vi "Find Direct Dependencies.vi"(8 "error in (no error)":errorcluster, 9 "LibraryName":string="ModuleA", 10 "Project Path":path=path "E:/sw-deps-monitor/Source/BuildSpecs/Modules/ModuleA.lvproj") -> (0 "error out":errorcluster, 2 "InDirect ActualDependencies":string[](array[string]), 3 "Direct ActualDependencies":string[](array[string]))   [LabVIEW 2019, in "Hawkeye.lvlib"]
uses:
  Hawkeye.lvlib
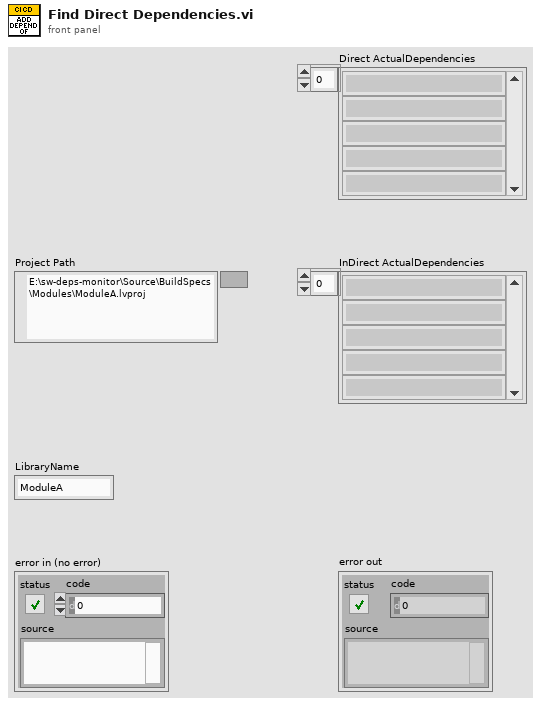
[diagram p1: front panel]
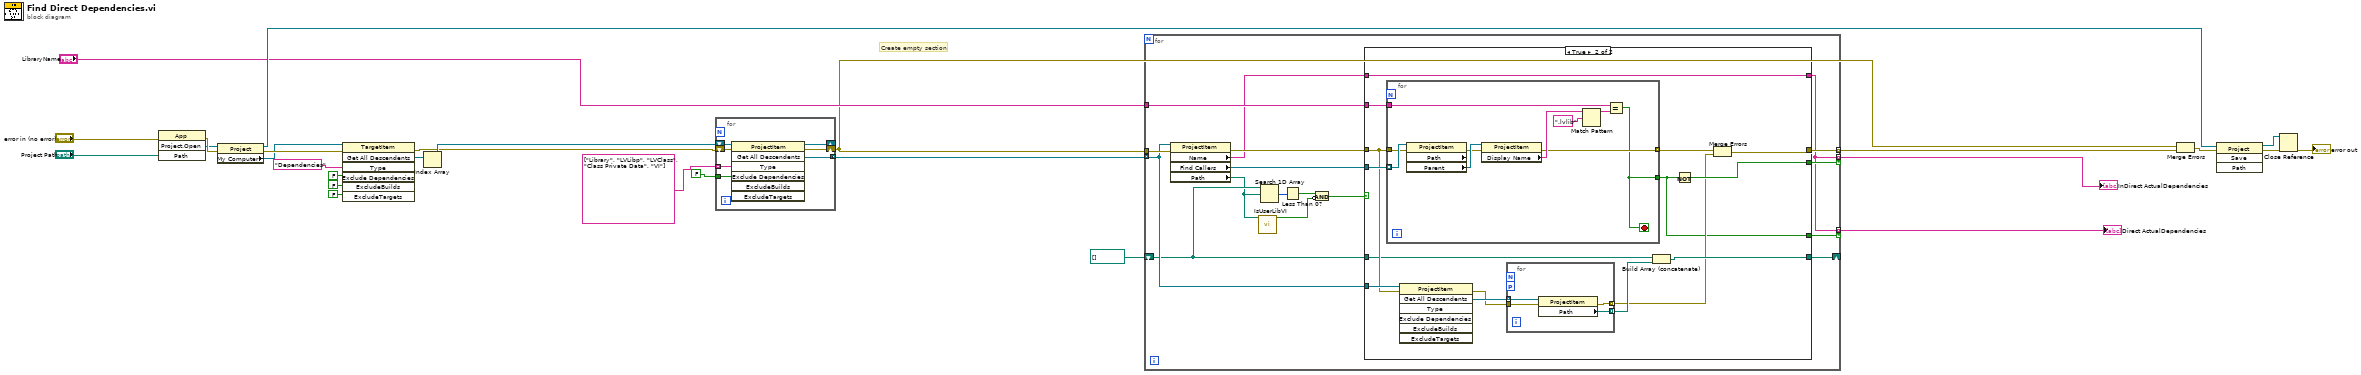
[diagram p0: block diagram]
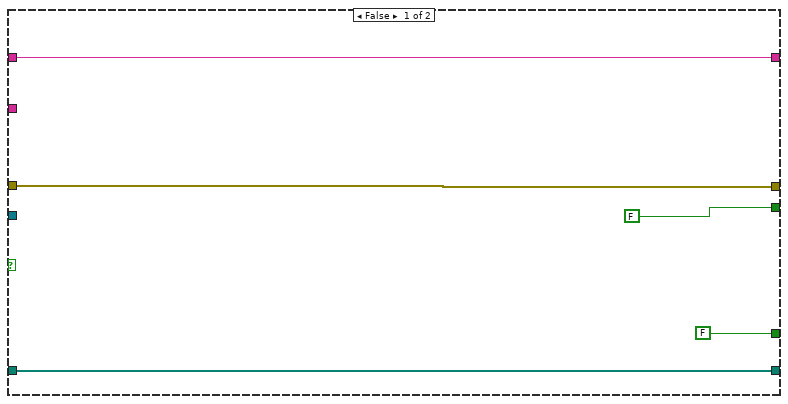
[diagram p2: hidden frame]
diagram:
  # "Create empty section"
  n1 = invoke class="App" method="Project.Open"(error in="error in (no error)", "Path"="Project Path") -> (error out=w26:errorcluster, "Project:Open"=w11:refnum<vi>)  [unwired: 2 in, 2 out]
  n2 = property class="Project"(reference=w11, error in=w26) -> (reference out=w17:refnum<vi>, error out=w20:errorcluster, "My Computer"=w10:refnum<vi>)
  n3 = invoke class="TargetItem" method="Get All Descendents"(reference=w10, error in=w20, "Type"="Dependencies", "Exclude Dependencies"=FALSE ("ExcludeDependencies"), "ExcludeBuilds"=FALSE, "ExcludeTargets"=FALSE) -> (error out=w19:errorcluster, "All Descendents"=w9:refnum<vi>[])  [unwired: 1 in, 5 out]
  n4 = Index Array(array=w9) -> (element=w21:refnum<vi>)  [unwired: 1 in]
  n5 = for {
    shift-right: [w33] -> _
    shift-left: w21 -> [w34]
    shift-right: [w31] -> w5
    shift-left: w19 -> [w32]
    tunnel: FALSE ("ExcludeDependencies") -> [w28]
    tunnel: string[] ["Library", "LVLibp", "LVClass", "Class Private Data", "VI"] ("Type") -> [w30] mode=indexing
    tunnel: [w29] -> w2 mode=concatenating
    n6 = invoke class="ProjectItem" method="Get All Descendents"(reference=w34, error in=w32, "Type"=w30, "Exclude Dependencies"=w28) -> (reference out=w33:refnum<vi>, error out=w31:errorcluster, "All Descendents"=w29:refnum<vi>[])  [unwired: 3 in, 4 out]
  }
  n7 = for {
    tunnel: w5 -> [w51]
    tunnel: w2 -> [w44] mode=indexing
    tunnel: "LibraryName" -> [w49]
    tunnel: [w43] -> w25 mode=indexing
    tunnel: [w40] -> w12 mode=indexing if=w46
    tunnel: [w40] -> w6 mode=indexing if=w48
    shift-right: [w47] -> _
    shift-left: path[] [] -> [w42]
    n8 = property class="ProjectItem"(reference=w44, error in=w51) -> (error out=w45:errorcluster, "Name"=w41:string, "Find Callers"=w50:refnum<vi>[], "Path"=w39:path)  [unwired: 1 out]
    n9 = call "IsUserLibVI.vi"("ItemPath"=w39) -> ("IsUserLibVI?"=w37:bool)  [unwired: 10 in]
    n10 = Search 1D Array(1D array=w42, element=w39) -> (index of element=w36:i32)  [unwired: 1 in]
    n11 = Less Than 0?(x=w36) -> (x < 0?=w38:bool)
    n12 = Compound Arithmetic op=AND(w38, invert w37) -> (w35:bool)
    n13 = case shown="True" w35 {
      tunnel: w50 -> [_ w71]
      tunnel: w49 -> [_ w70]
      tunnel: [FALSE w57] -> w48
      tunnel: [w55 w68] -> w47
      tunnel: w42 -> [w55 w59]
      tunnel: [FALSE w67] -> w46
      tunnel: w45 -> [w53 w60]
      tunnel: w44 -> [_ w65]
      tunnel: [w53 w62] -> w43
      tunnel: w41 -> [w52 w58]
      tunnel: [w52 w58] -> w40
      frame False {
      }
      frame True {
        n14 = for {
          tunnel: w71 -> [w85] mode=indexing
          tunnel: w70 -> [w77]
          tunnel: [w80] -> w57
          tunnel: [w81] -> w63 mode=indexing
          tunnel: w60 -> [w79]
          stop <- w80 stop-if-true
          n15 = property class="ProjectItem" props=["Path", "Parent"](reference=w85, error in=w79) -> (error out=w78:errorcluster, "Parent"=w84:refnum<vi>)  [unwired: 2 out]
          n16 = property class="ProjectItem"(reference=w84, error in=w78) -> (error out=w81:errorcluster, "Display Name"=w82:string)  [unwired: 1 out]
          n17 = Match Pattern(string=w82, regular expression=".lvlib") -> (before substring=w76:string)  [unwired: 1 in, 3 out]
          n18 = Equal?(x=w77, y=w76) -> (x = y?=w80:bool)
        }
        n19 = invoke class="ProjectItem" method="Get All Descendents"(reference=w65, error in=w60) -> (error out=w64:errorcluster, "All Descendents"=w66:refnum<vi>[])  [unwired: 5 in, 5 out]
        n20 = for {
          tunnel: w66 -> [w75] mode=indexing
          tunnel: [w74] -> w69 mode=indexing
          tunnel: w64 -> [w73]
          tunnel: [w72] -> w61 mode=indexing
          workers-P: _ -> [_]
          n21 = property class="ProjectItem"(reference=w75, error in=w73) -> (error out=w72:errorcluster, "Path"=w74:path)  [unwired: 1 out]
        }
        n22 = Build Array (concatenate)(w59, w69) -> (w68:path[])
        n23 = Not(x=w57) -> (.not. x?=w67:bool)
        n24 = Merge Errors(w63, w61) -> (w62:errorcluster)
      }
    }
  }
  "InDirect ActualDependencies" <- w12
  "Direct ActualDependencies" <- w6
  n25 = Merge Errors(w5, w25) -> (w18:errorcluster)
  n26 = invoke class="Project" method="Save"(reference=w17, error in=w18) -> (reference out=w16:refnum<vi>, error out=w15:errorcluster)  [unwired: 2 in, 2 out]
  n27 = Close Reference(reference=w16, error in (no error)=w15) -> (error out=→"error out":errorcluster)
